vi "Logger.vi"() -> ()   [LabVIEW 2017]
panel:
  out "Temperature":cluster{timestamp[], dbl[]}(graph)
  out "ADC Counts":cluster{timestamp[], i32[]}(graph)
  in  "File Path":path
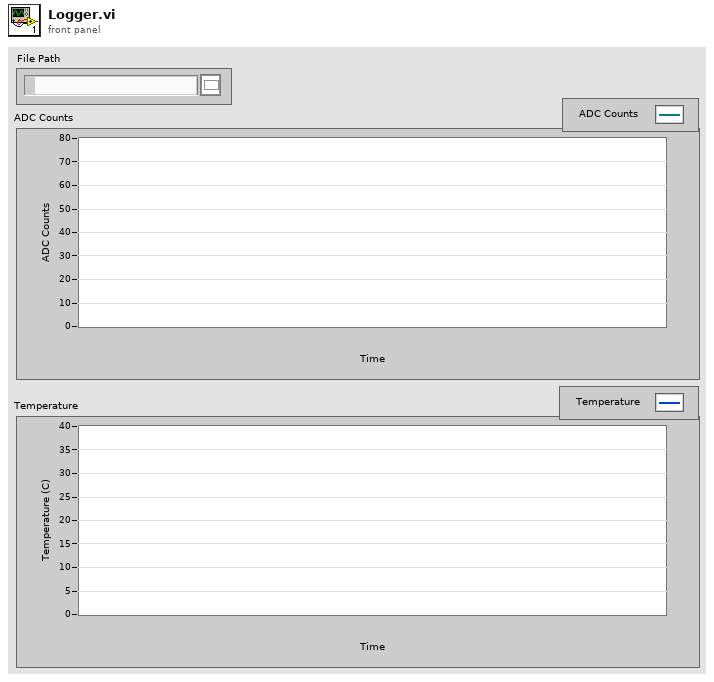
[diagram p1: front panel]
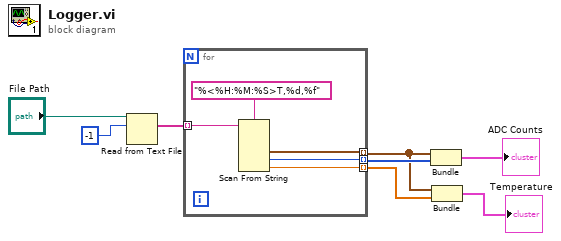
[diagram p0: block diagram]
diagram:
  n1 = Read from Text File(file (use dialog)="File Path", count=-1) -> (text=w8:string[])  [unwired: 2 in, 3 out]
  n2 = for {
    tunnel: w8 -> [w13] mode=indexing
    tunnel: [w10] -> w3 mode=indexing
    tunnel: [w11] -> w7 mode=indexing
    tunnel: [w9] -> w2 mode=indexing
    n3 = Scan From String(format string="%<%H:%M:%S>T,%d,%f", input string=w13) -> (output 1=w10:timestamp, output 2=w11:i32, output 3=w9:dbl)  [unwired: 5 in, 3 out]
  }
  n4 = Bundle(w3, w7) -> (→"ADC Counts":cluster{timestamp[], i32[]})  [unwired: 1 in]
  n5 = Bundle(w3, w2) -> (→"Temperature":cluster{timestamp[], dbl[]})  [unwired: 1 in]
